vi "activate autocomplete v2.vi"(5 "BluePlotHandle in":refnum<class "RocketPlotHandle.lvclass">, 7 "Refs":T1, 8 "error in (no error)":errorcluster, 9 "Flatline?":bool, 10 "Index":i32) -> (0 "error out":errorcluster)   [LabVIEW 2021, in "RocketPlot.lvlib"]
uses:
  RocketPlot.lvlib
  TypeDefs/Plot UI references.ctl
  Classes/RocketPlotHandle/RocketPlotHandle.lvclass
  <userlib>/bjustice/TipStripOOPanel/Classes/TipPanelHandle/TipPanelHandle.lvclass
  TypeDefs/Plot top row.ctl
  Autocomplete popup/subvis/input options.ctl
  <vilib>/Utility/miscctls.llb/LVPointTypeDef.ctl
  Autocomplete popup/Autocomplete popup.lvlib
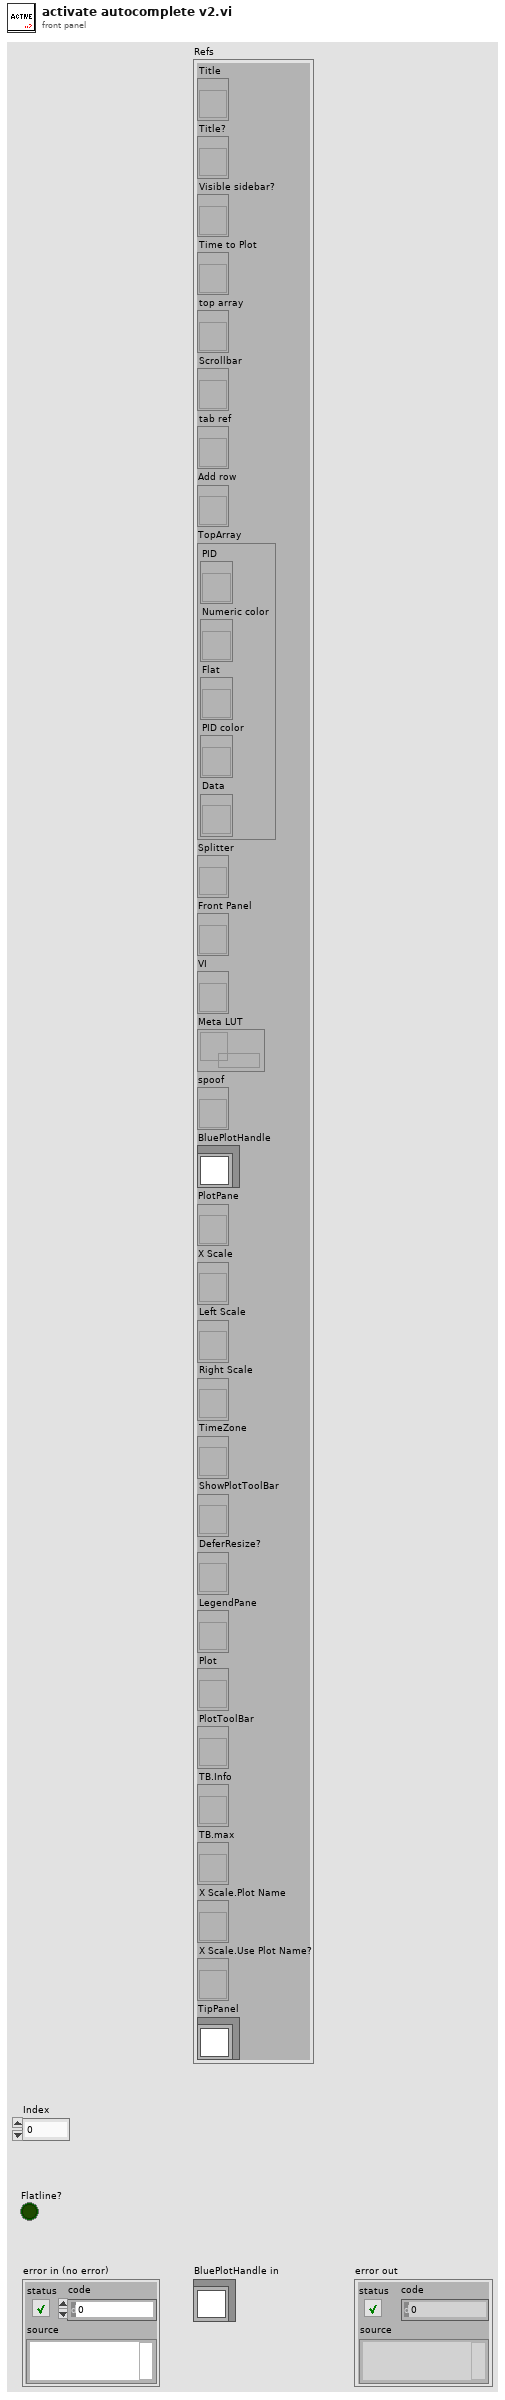
[diagram p1: front panel]
types:
  T1 = typedef "RocketPlot.lvlib/Plot UI references.ctl" = cluster{"Title":refnum<vi>, "Title?":refnum<vi>, "Visible sidebar?":refnum<vi>, "Time to Plot":refnum<vi>, "top array":refnum<vi>, "Scrollbar":refnum<vi>, "tab ref":refnum<vi>, "Add row":refnum<vi>, "TopArray":cluster{"PID":refnum<vi>, "Numeric color":refnum<vi>, "Flat":refnum<vi>, "PID color":refnum<vi>, "Data":refnum<vi>}, "Splitter":refnum<vi>, "Front Panel":refnum<vi>, "VI":refnum<vi>, "Meta LUT":refnum<data-value>, "spoof":refnum<vi>, "BluePlotHandle":refnum<class "RocketPlotHandle.lvclass">, "PlotPane":refnum<vi>, "X Scale":refnum<vi>, "Left Scale":refnum<vi>, "Right Scale":refnum<vi>, "TimeZone":refnum<vi>, "ShowPlotToolBar":refnum<vi>, "DeferResize?":refnum<vi>, "LegendPane":refnum<vi>, "Plot":refnum<vi>, "PlotToolBar":refnum<vi>, "TB.Info":refnum<vi>, "TB.max":refnum<vi>, "X Scale.Plot Name":refnum<vi>, "X Scale.Use Plot Name?":refnum<vi>, "TipPanel":refnum<class "TipPanelHandle.lvclass">}
  T2 = typedef "Autocomplete popup.lvlib/input options.ctl" = cluster{"Screen Coordinates":T3, "Width":u32, "max rows":i32, "List":string[], "init value":string}
  T3 = typedef "LVPointTypeDef.ctl" = cluster{"Horizontal":i16, "Vertical":i16}
  T4 = typedef "LVPositionTypeDef.ctl" = cluster{"Left":i32, "Top":i32}
  T5 = typedef "Plot top row.ctl" = cluster{"PID":string, "index":i32, "PID color":u32, "right axis?":bool, "Flatline?":bool, "Numeric color":u32, "Data":string, "Flat":string}
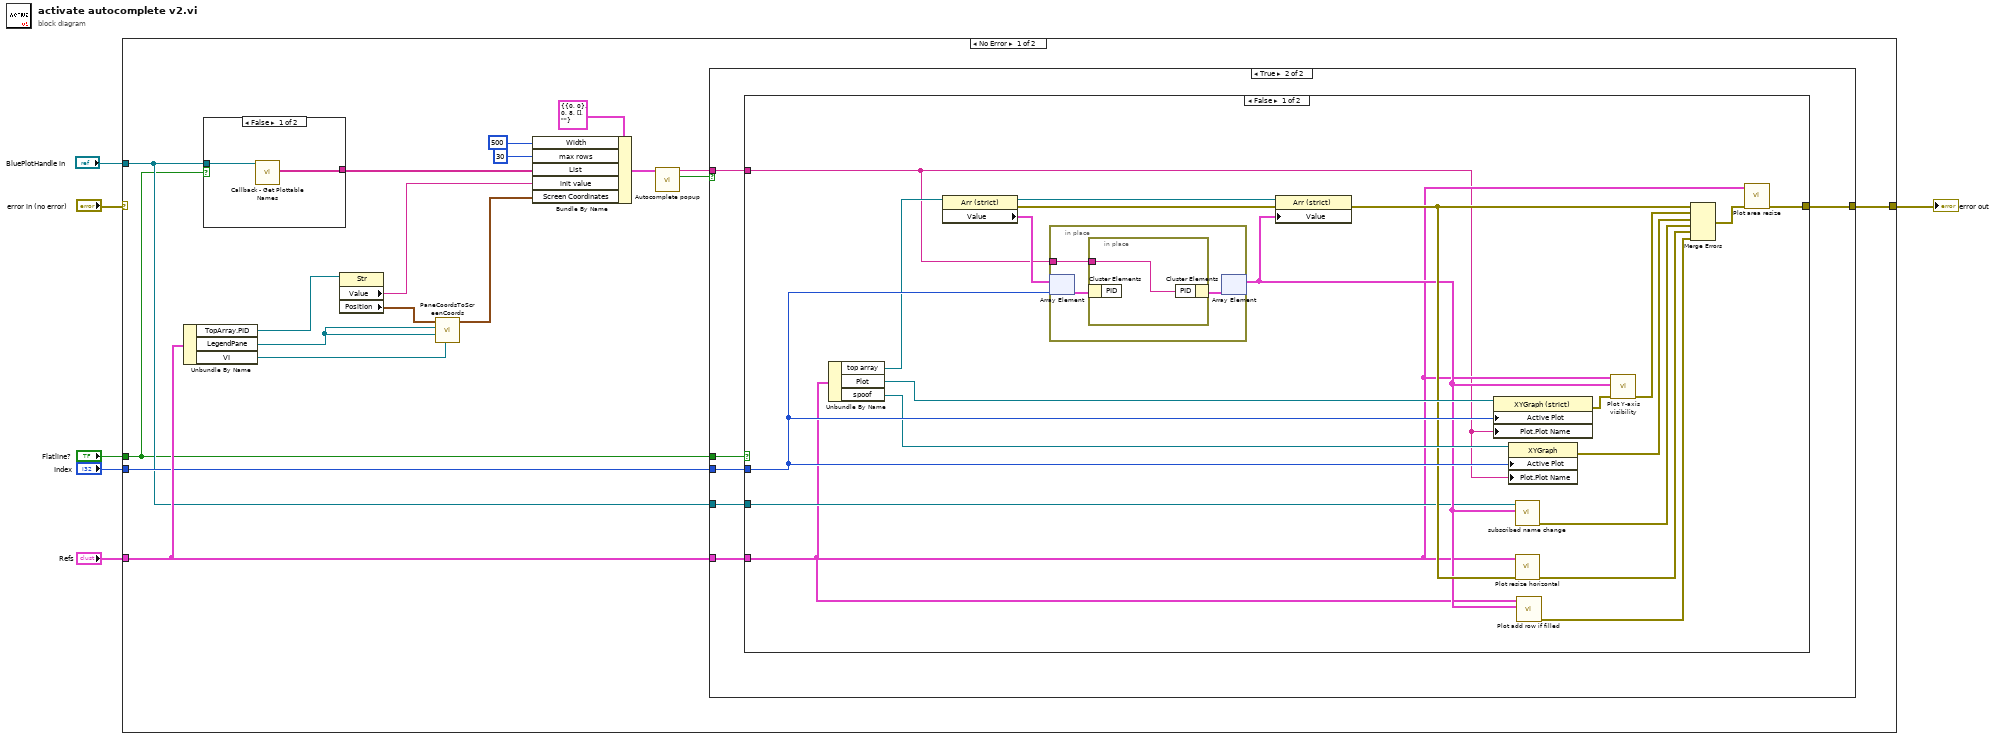
[diagram p0: block diagram]
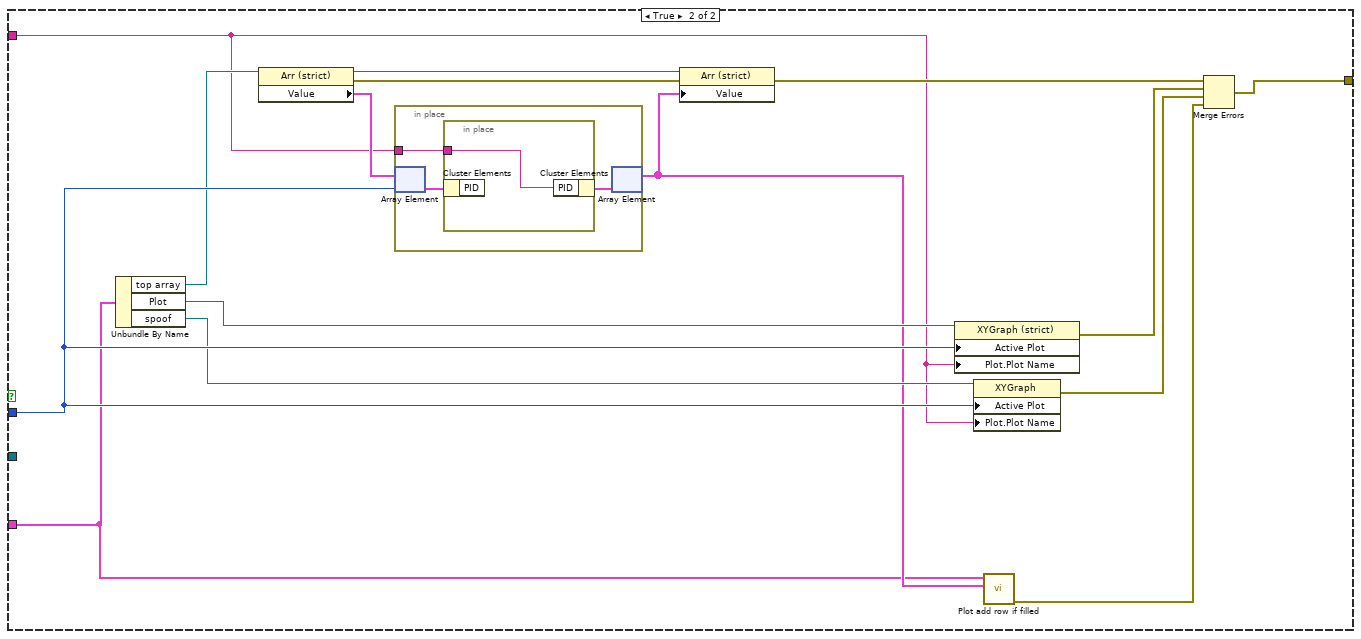
[diagram p4: hidden frame]
diagram:
  n1 = case shown="No Error" "error in (no error)" {
    selector: "error in (no error)" -> [_ w76]
    tunnel: "Refs" -> [w16 _]
    tunnel: [w13 w76] -> w5
    tunnel: "Index" -> [w15 _]
    tunnel: "Flatline?" -> [w11 _]
    tunnel: "BluePlotHandle in" -> [w14 _]
    frame No Error {
      n2 = Unbundle By Name(w16) -> ("TopArray.PID"=w12:refnum<vi>, "LegendPane"=w9:refnum<vi>, "VI"=w8:refnum<vi>)
      n3 = case shown="False" w11 {
        tunnel: [w26 _] -> w20
        tunnel: w14 -> [w25 _]
        frame False {
          n4 = call-dynamic "Callback - Get Plottable Names.vi"("BluePlotHandle in"=w25) -> ("Plottable Names"=w26:string[])  [unwired: 8 in, 2 out]
        }
        frame True {
        }
      }
      n5 = property on="Property Node" class="Str"(reference=w12) -> ("Value"=w21:string, "Position"=w10:T4)  [unwired: 1 in, 2 out]
      n6 = call "PaneCoordsToScreenCoords.vi"("VI"=w8, "Origin Pane"=w9, "Owning Pane"=w9, "Pane Coordinates"=w10) -> ("Screen Coords"=w7:T3)  [unwired: 6 in, 1 out]
      n7 = Bundle By Name(cluster=T2 {"Screen Coordinates"={"Horizontal"=0, "Vertical"=0}, "Width"=0, "max rows"=8, "List"=[], "init value"=""} ("input"), "Width"=u32 500, "max rows"=30, "List"=w20, "init value"=w21, "Screen Coordinates"=w7) -> (w19:T2)
      n8 = call "Autocomplete popup.vi"("input"=w19) -> ("Accept?"=w18:bool, "String"=w17:string)  [unwired: 8 in, 1 out]
      n9 = case shown="True" w18 {
        tunnel: w17 -> [_ w30]
        tunnel: w11 -> [_ w32]
        tunnel: w16 -> [_ w31]
        tunnel: w15 -> [_ w29]
        tunnel: w14 -> [_ w28]
        tunnel: [_ w27] -> w13
        frame False {
        }
        frame True {
          n10 = case shown="False" w32 {
            tunnel: w29 -> [w52 w71]
            tunnel: [w39 w58] -> w27
            tunnel: w28 -> [w40 _]
            tunnel: w31 -> [w37 w63]
            tunnel: w30 -> [w33 w59]
            frame False {
              n11 = Unbundle By Name(w37) -> ("top array"=w45:refnum<vi>, "Plot"=w48:refnum<vi>, "spoof"=w47:refnum<vi>)
              n12 = property class="Arr (strict)"(reference=w45) -> (reference out=w35:refnum<vi>, error out=w34:errorcluster, "Value"=w36:T5[])  [unwired: 1 in]
              n13 = in-place {
                in-place-border: w33 -> [w54]
                n14 = in-place-array #1(w36, w52) -> (w55:T5)
                n15 = in-place {
                  in-place-border: w54 -> [w56]
                  n16 = in-place-cluster #2(w55) -> ()  [unwired: 1 out]
                  n17 = in-place-cluster #2("PID"=w56) -> (w53:T5)
                }
                n18 = in-place-array #1(w53) -> (w41:T5[])  [unwired: 1 out]
              }
              n19 = property class="Arr (strict)"(reference=w35, error in=w34, "Value"=w41) -> (error out=w43:errorcluster)  [unwired: 1 out]
              n20 = property class="XYGraph (strict)"(reference=w48, "Active Plot"=w52, "Plot.Plot Name"=w33) -> (error out=w50:errorcluster)  [unwired: 1 in, 1 out]
              n21 = property class="XYGraph"(reference=w47, "Active Plot"=w52, "Plot.Plot Name"=w33) -> (error out=w51:errorcluster)  [unwired: 1 in, 1 out]
              n22 = call "subscribed name change.vi"("top array"=w41, "BluePlotHandle"=w40) -> ("error out"=w42:errorcluster)  [unwired: 9 in]
              n23 = call "Plot resize horizontal.vi"("error in (no error)"=w43, "Refs"=w37) -> ("error out"=w46:errorcluster)  [unwired: 9 in]
              n24 = call "Plot add row if filled.vi"("top array"=w41, "Refs"=w37) -> ("error out"=w44:errorcluster)  [unwired: 8 in, 1 out]
              n25 = call "Plot Y-axis visibility.vi"("error in (no error)"=w50, "top array"=w41, "Refs"=w37) -> ("error out"=w49:errorcluster)  [unwired: 8 in]
              n26 = Merge Errors(w43, w49, w51, w42, w46, w44) -> (w38:errorcluster)
              n27 = call "Plot area resize.vi"("error in (no error)"=w38, "Refs"=w37) -> ("error out"=w39:errorcluster)  [unwired: 9 in]
            }
            frame True {
              n28 = Unbundle By Name(w63) -> ("top array"=w67:refnum<vi>, "Plot"=w69:refnum<vi>, "spoof"=w68:refnum<vi>)
              n29 = property class="Arr (strict)"(reference=w67) -> (reference out=w61:refnum<vi>, error out=w60:errorcluster, "Value"=w62:T5[])  [unwired: 1 in]
              n30 = in-place {
                in-place-border: w59 -> [w73]
                n31 = in-place-array #3(w62, w71) -> (w74:T5)
                n32 = in-place {
                  in-place-border: w73 -> [w75]
                  n33 = in-place-cluster #4(w74) -> ()  [unwired: 1 out]
                  n34 = in-place-cluster #4("PID"=w75) -> (w72:T5)
                }
                n35 = in-place-array #3(w72) -> (w64:T5[])  [unwired: 1 out]
              }
              n36 = property class="Arr (strict)"(reference=w61, error in=w60, "Value"=w64) -> (error out=w65:errorcluster)  [unwired: 1 out]
              n37 = property class="XYGraph (strict)"(reference=w69, "Active Plot"=w71, "Plot.Plot Name"=w59) -> (error out=w57:errorcluster)  [unwired: 1 in, 1 out]
              n38 = property class="XYGraph"(reference=w68, "Active Plot"=w71, "Plot.Plot Name"=w59) -> (error out=w70:errorcluster)  [unwired: 1 in, 1 out]
              n39 = call "Plot add row if filled.vi"("top array"=w64, "Refs"=w63) -> ("error out"=w66:errorcluster)  [unwired: 8 in, 1 out]
              n40 = Merge Errors(w65, w57, w70, w66) -> (w58:errorcluster)
            }
          }
        }
      }
    }
    frame Error {
    }
  }
  "error out" <- w5
